vi "Editor.vi"(8 "error in (no error)":errorcluster, 10 "Browse start path":path caption="start path") -> (0 "error out":errorcluster, 3 "Uncompiled sequence out":T2[](array[typedef]))   [LabVIEW 2020, in "Sequencer.lvlib"]
doc: "Sequence editor used to configure, save and load sequences put together of messages."
uses:
  Sequencer.lvlib
  Controls/Ctl_SequenceElement.ctl
  Controls/Ctl_SequenceControlElement.ctl
  PPL/HDH.Actor Framework.Core.Msg.lvlibp/Flex Msg/Controls/Ctl_Control Element.ctl
  Controls/Ctl_MessageListElement.ctl
  PPL/HDH.Actor Framework.Core.Msg.lvlibp/Flex Msg/Flex Msg.lvclass
  PPL/HDH.Actor Framework.Core.Msg.lvlibp
panel:
  in  "Refresh Class List":bool
  in  "Tab Control":T1(tab)
  in  "Message List":i32(listbox)
  in  "Hierarchy Tree":string(tree)
  in  "Search List":i32(listbox)
  in  "Message Filter":string
  in  "Load":bool
  in  "Save":bool
  in  "Append":bool
  in  "Insert":bool
  in  "Sequence":i32[](listbox)
  in  "Empty":bool
  in  "Done":bool
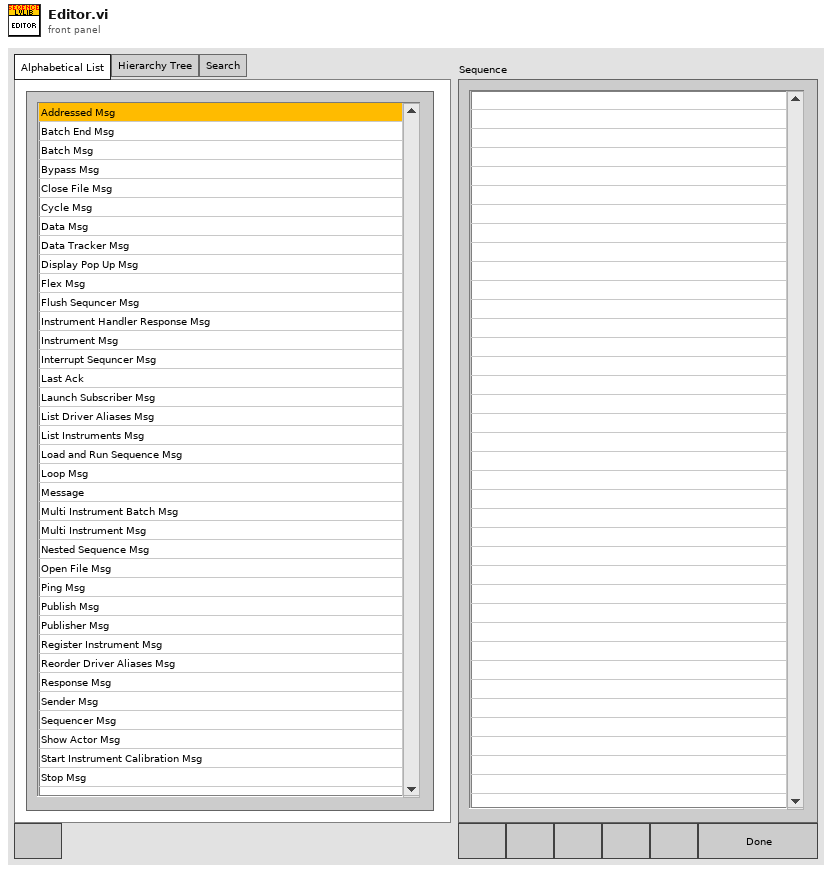
[diagram p1: front panel]
types:
  T1 = enum32{"Alphabetical List", "Hierarchy Tree", "Search"}
  T2 = typedef "Sequencer.lvlib/Ctl_SequenceElement.ctl" = cluster{"Message Base Name":string, "Message Path":path, "Supports Data Access?":bool, "List Symbol":i32, "Sequence Control Element Array":T3[]}
  T3 = typedef "Sequencer.lvlib/Ctl_SequenceControlElement.ctl" = cluster{"Data Override name":string, "Looped Override?":bool, "Control element":T4, "List Symbol":i32}
  T4 = typedef "HDH.Actor Framework.Core.Msg.lvlibp/Ctl_Control Element.ctl" = cluster{"Index":i32, "Label":string, "Value":variant}
  T5 = typedef "Sequencer.lvlib/Ctl_MessageListElement.ctl" = cluster{"Base Name":string, "List index":i32, "Msg path":path, "Supports DA?":bool, "Symbol":i32}
  T6 = typedef "eventvkey.ctl" = enum16{"ASCII", "Enter", "Return", "Shift", "Ctrl", "Alt", "Cmd", "Opt", "Caps", "NumLock", "Clear", "Break", "Up", "Down", "Left", "Right", "Insert", "Delete", "Home", "End", "PageUp", "PageDown", "Escape", "Help", "Pause", "ScrollLock", "F1", "F2", "F3", "F4", "F5", "F6", "F7", "F8", "F9", "F10", "F11", "F12", "F13", "F14", "F15", "F16", "F17", "F18", "F19", "F20", "F21", "F22", "F23", "F24", "Play", "VolumeUp", "VolumeDown", "Mute", "Two Byte Char"}
  T7 = typedef "lveventtype.ctl" = enum32{"Null", "Timeout", "Annotation Menu Selection", "Annotation Menu Selection?", "App Instance Close", "App Instance Close?", "Autoscale Range Change", "Bookmark Info Change", "Cell Edit", "Cell Edit?", "Cursor Grab", "Cursor Grab?", "Cursor Menu Selection", "Cursor Menu Selection?", "Cursor Move", "Cursor Release", "Data Change", "Direction Change", "Display State Change", "Drag Ended", "Drag Enter", "Drag Leave", "Drag Over", "Drag Source Update", "Drag Starting", "Drag Starting?", "Drop", "Exec State Change", "Key Down", "Key Down?", "Key Repeat", "Key Repeat?", "Key Up", "Listbox Double Click", "Menu Activation?", "Menu Selection (App)", "Menu Selection? (App)", "Menu Selection (User)", "Mouse Down", "Mouse Down?", "Mouse Enter", "Mouse Leave", "Mouse Move", "Mouse Up", "Mouse Wheel", "NI Security User Change (App)", "Pane Size", "Panel Close", "Panel Close?", "Panel Resize", "Plot Attribute Change", "Scale Range Change", "Shortcut Menu Activation?", "Shortcut Menu Selection (App)", "Shortcut Menu Selection? (App)", "Shortcut Menu Selection (User)", "Tree Double Click", "Tree Drag", "Tree Drag?", "Tree Drop", "Tree Drop?", "Tree Item Close", "Tree Item Close?", "Tree Item Open", "Tree Item Open?", "User Event", "Value Change"}
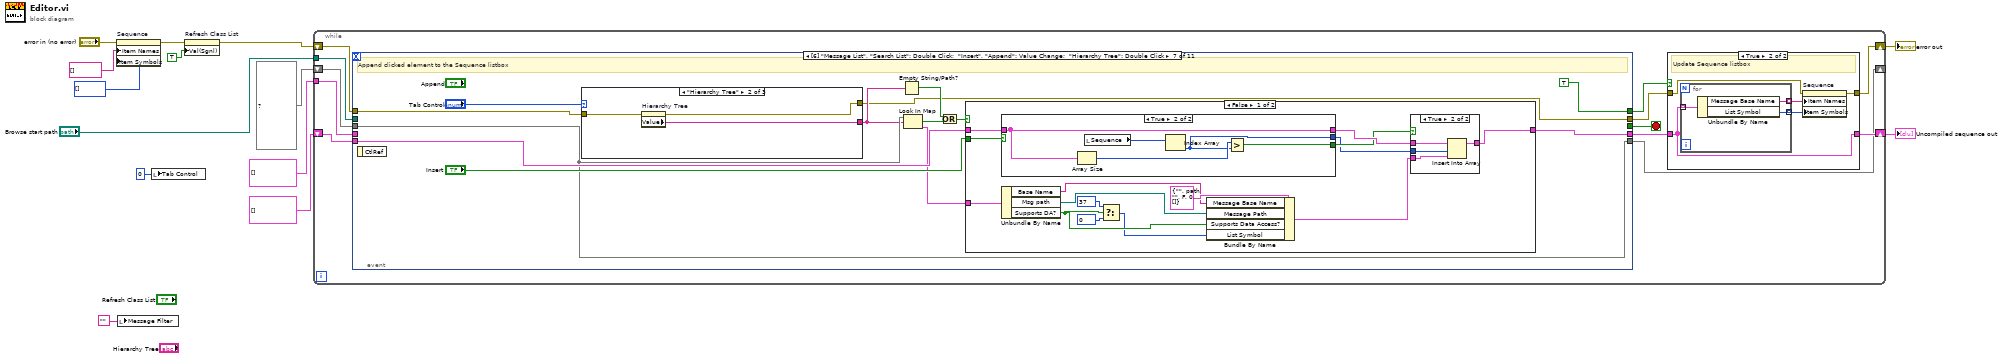
[diagram p0: block diagram]
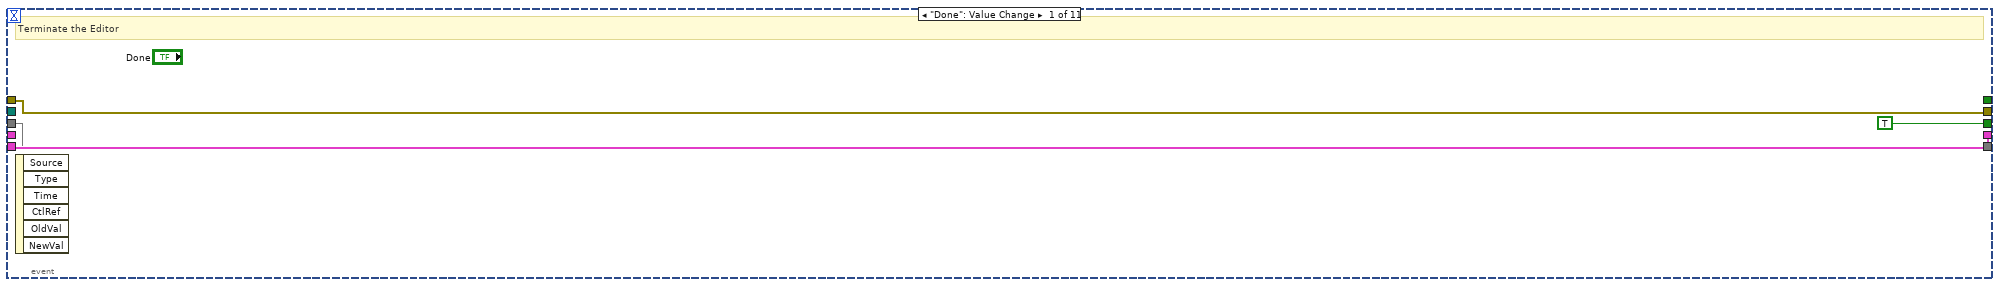
[diagram p3: hidden frame]
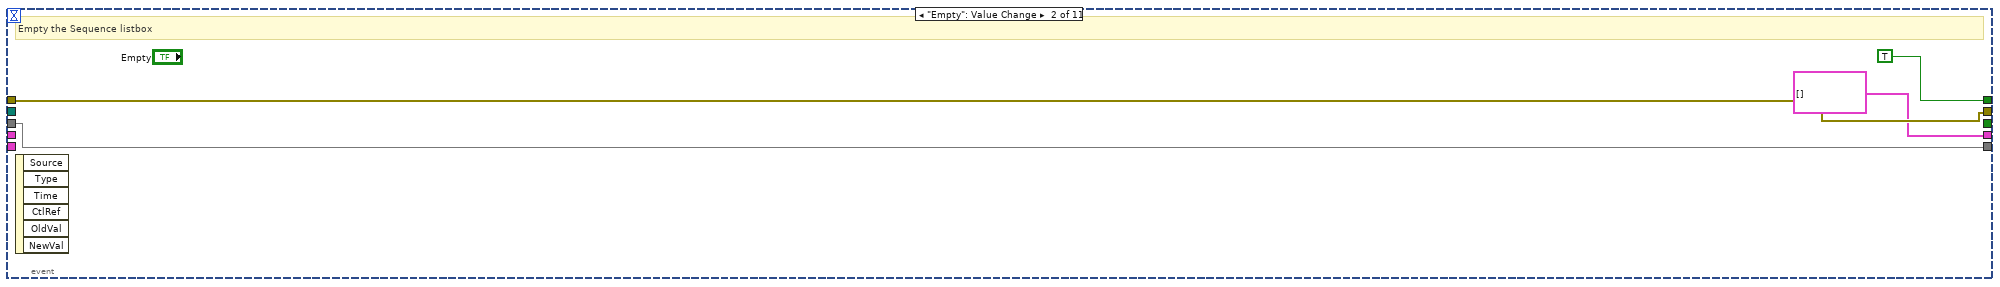
[diagram p4: hidden frame]
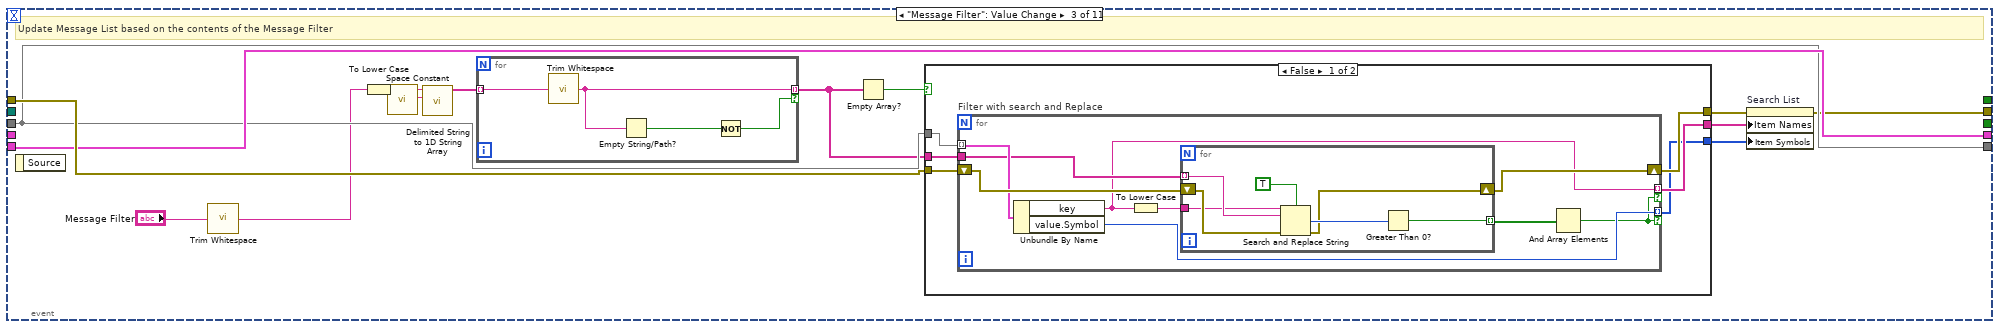
[diagram p5: hidden frame]
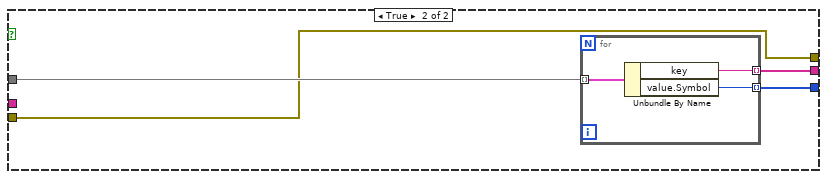
[diagram p6: hidden frame]
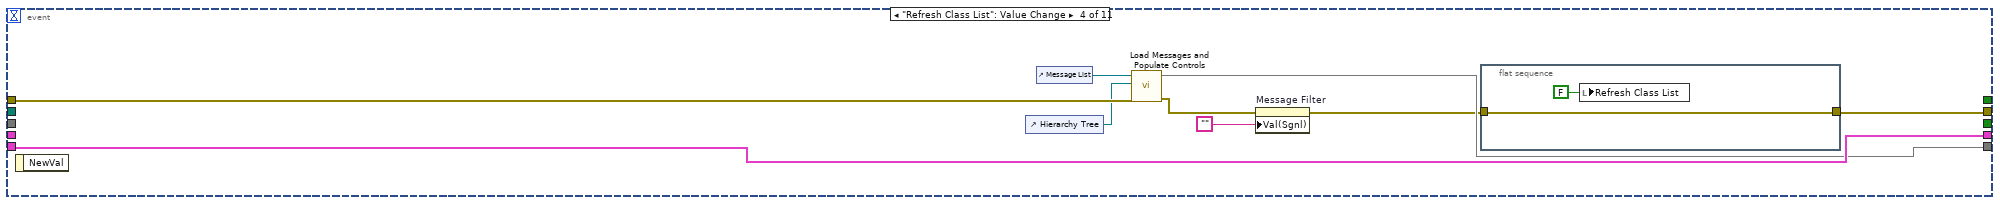
[diagram p7: hidden frame]
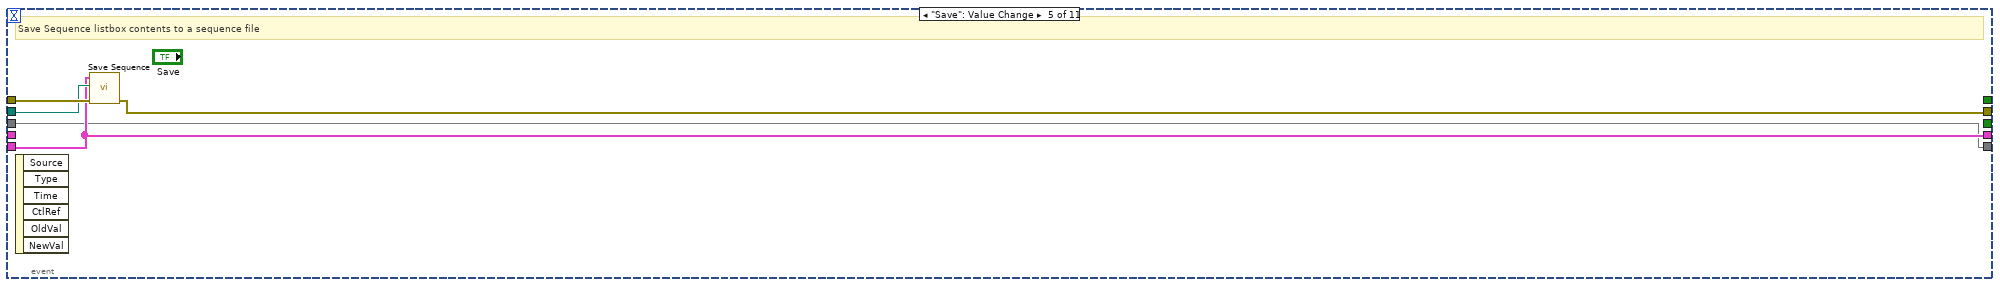
[diagram p8: hidden frame]
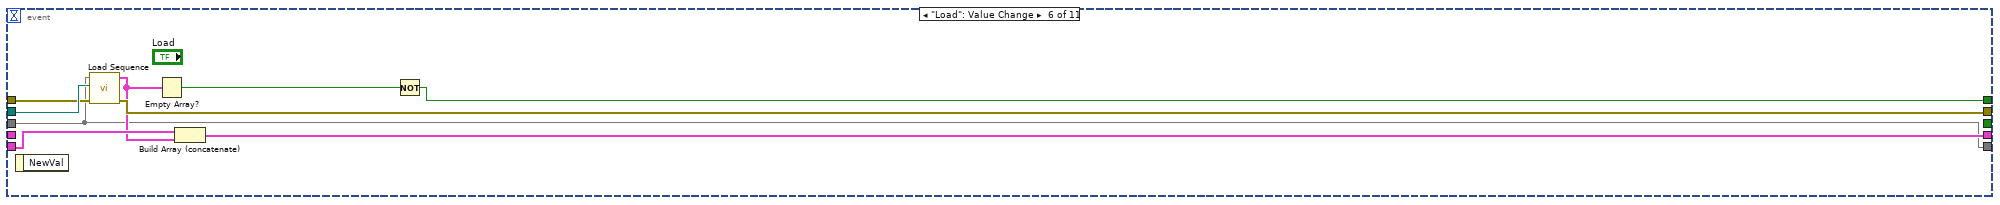
[diagram p9: hidden frame]
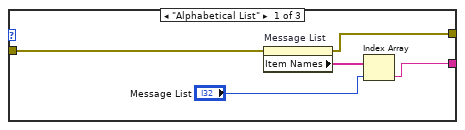
[diagram p10: hidden frame]
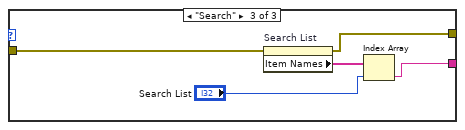
[diagram p11: hidden frame]
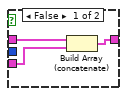
[diagram p12: hidden frame]
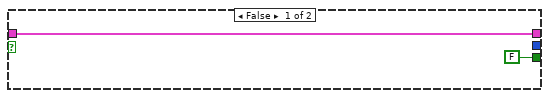
[diagram p13: hidden frame]
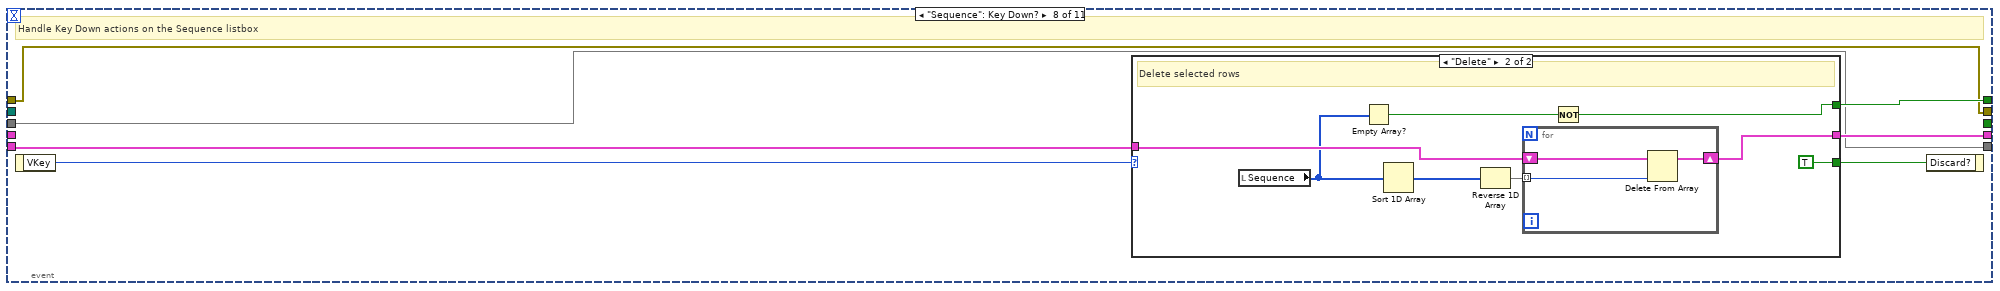
[diagram p15: hidden frame]
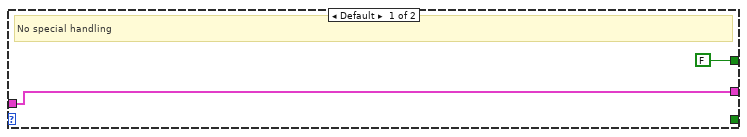
[diagram p16: hidden frame]
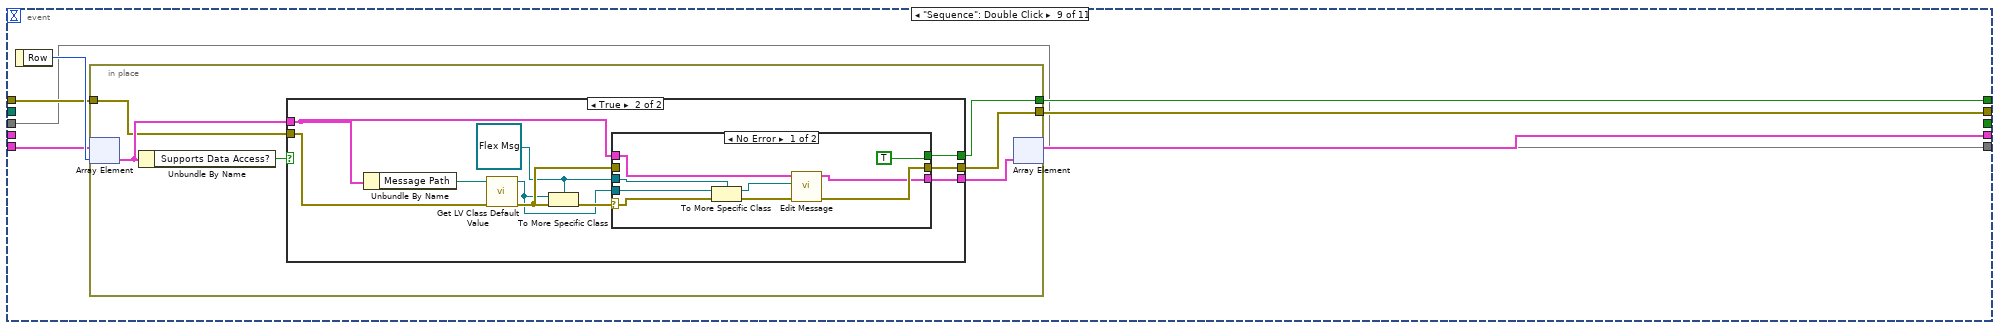
[diagram p17: hidden frame]
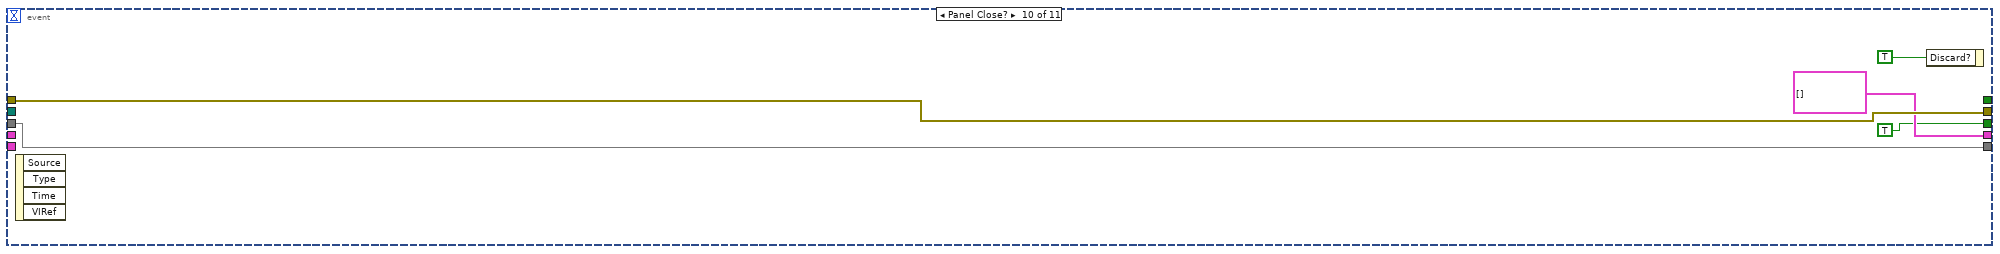
[diagram p20: hidden frame]
diagram:
  n1 = property on="Sequence" class="LstBox (strict)"(error in="error in (no error)", "Item Names"=string[] [], "Item Symbols"=i32[] []) -> (error out=w4:errorcluster)  [unwired: 1 in, 1 out]
  n2 = local write "Message Filter"("") -> ()
  n3 = local write "Tab Control"(u32 0) -> ()
  n4 = property on="Refresh Class List" class="Bool (strict)"(error in=w4, "Val(Sgnl)"=TRUE) -> (error out=w7:errorcluster)  [unwired: 1 in, 1 out]
  n5 = while {
    shift-right: [w19] -> w10
    shift-left: w7 -> [w25]
    shift-right: [w21] -> w11
    shift-left: T2[] [] ("Uncompiled sequence in") -> [w24]
    tunnel: "Browse start path" -> [w18]
    tunnel: T4[] [] ("Control Element Array") -> [w17]
    shift-right: [w15] -> _
    shift-left: map{string, T5} {} ("map") -> [w16]
    stop <- w26 stop-if-true
    n6 = event shown="[6] \"Message List\", \"Search List\": Double Click;  \"Insert\", \"Append\": Value Change;  \"Hierarchy Tree\": Double Click" {
      selector: _ -> [_ _ _ _ _ _ _ _ _ _ _]
      dyn-events: _ -> [_ _ _ _ _ _ _ _ _ _ _]
      timeout: _ -> [_ _ _ _ _ _ _ _ _ _ _]
      tunnel: [TRUE _ _ _ _ _ _ _ _ TRUE _] -> w26
      tunnel: [w39 w44 w53 w99 w106 w112 w118 w174 w195 w233 w243] -> w20
      tunnel: w25 -> [w39 w44 w58 w98 w107 w113 w117 w174 w196 w233 w243]
      tunnel: [w38 T2[] [] ("Uncompiled sequence in") w57 w100 w104 w114 w128 w177 w197 T2[] [] ("Uncompiled sequence in") w237] -> w22
      tunnel: w24 -> [w38 _ w57 w100 w104 w115 w129 w178 w198 _ w238]
      tunnel: [_ TRUE _ _ _ w109 TRUE w176 w194 _ w235] -> w23
      tunnel: w18 -> [_ _ _ _ w105 w116 _ _ _ _ _]
      tunnel: w17 -> [_ _ _ _ _ _ _ _ _ _ _]
      tunnel: w16 -> [w37 w41 w56 _ w103 w108 w124 w173 w193 w229 w234]
      tunnel: [w37 w41 w56 w96 w103 w108 w124 w173 w193 w229 w234] -> w15
      event "Done": Value Change {
        # "Terminate the Editor"
        n7 = event-data() -> ()  [unwired: 1 in, 6 out]
      }
      event "Empty": Value Change {
        # "Empty the Sequence listbox"
        n8 = event-data() -> ()  [unwired: 1 in, 6 out]
      }
      event "Message Filter": Value Change {
        # "Update Message List based on the contents of the Message Filter"
        n9 = event-data() -> ()  [unwired: 1 in, 1 out]
        n10 = call <vilib>:"Trim Whitespace.vi"("string"="Message Filter") -> ("trimmed string"=w52:string)  [unwired: 1 in]
        n11 = To Lower Case(string=w52) -> (all lower case string=w51:string)
        n12 = call <vilib>:"Space Constant.vi"() -> ("String"=w50:string)
        n13 = call <vilib>:"Delimited String to 1D String Array.vi"("delimiter"=w50, "delimited string"=w51) -> ("string array"=w49:string[])  [unwired: 9 in]
        n14 = for {
          tunnel: w49 -> [w62] mode=indexing
          tunnel: [w61] -> w47 mode=indexing if=w59
          n15 = call <vilib>:"Trim Whitespace.vi"("string"=w62) -> ("trimmed string"=w61:string)  [unwired: 1 in]
          n16 = Empty String/Path?(string/path=w61) -> (empty?=w60:bool)
          n17 = Not(x=w60) -> (.not. x?=w59:bool)
        }
        n18 = Empty Array?(array=w47) -> (empty?=w48:bool)
        n19 = case shown="False" w48 {
          tunnel: [w67 w85] -> w46
          tunnel: w58 -> [w68 w85]
          tunnel: w56 -> [w66 w88]
          tunnel: [w64 w87] -> w55
          tunnel: [w63 w86] -> w54
          tunnel: w47 -> [w65 _]
          frame False {
            n20 = for "Filter with search and Replace" {
              tunnel: w66 -> [w76] mode=indexing
              tunnel: [w71] -> w64 mode=indexing if=w69
              shift-right: [w74] -> w67
              shift-left: w68 -> [w77]
              tunnel: w65 -> [w72]
              tunnel: [w70] -> w63 mode=indexing if=w69
              n21 = Unbundle By Name(w76) -> ("key"=w71:string, "value.Symbol"=w70:i32)
              n22 = To Lower Case(string=w71) -> (all lower case string=w73:string)
              n23 = for {
                tunnel: w72 -> [w83] mode=indexing
                tunnel: [w80] -> w75 mode=indexing
                tunnel: w73 -> [w78]
                shift-right: [w79] -> w74
                shift-left: w77 -> [w84]
                n24 = Search and Replace String(case sensitive?=TRUE ("ignore case? (F)"), input string=w78, search string=w83, error in=w84) -> (number of replacements=w81:i32, error out=w79:errorcluster)  [unwired: 4 in, 2 out]
                n25 = Greater Than 0?(x=w81) -> (x > 0?=w80:bool)
              }
              n26 = And Array Elements(Boolean array=w75) -> (logical AND=w69:bool)
            }
          }
          frame True {
            n27 = for {
              tunnel: w88 -> [w91] mode=indexing
              tunnel: [w90] -> w87 mode=indexing
              tunnel: [w89] -> w86 mode=indexing
              n28 = Unbundle By Name(w91) -> ("key"=w90:string, "value.Symbol"=w89:i32)
            }
          }
        }
        n29 = property on="Search List" class="LstBox (strict)"(error in=w46, "Item Names"=w55, "Item Symbols"=w54) -> (error out=w53:errorcluster)  [unwired: 1 in, 1 out]
      }
      event "Refresh Class List": Value Change {
        n30 = event-data() -> ()  [unwired: 1 in, 1 out]
        n31 = control-ref of="Hierarchy Tree"() -> (w95:refnum<vi>)
        n32 = control-ref of="Message List"() -> (w97:refnum<vi>)
        n33 = call "Load Messages and Populate Controls.vi"("error in (no error)"=w98, "Hierarchy"=w95, "ListBox in"=w97) -> ("error out"=w93:errorcluster, "Message map"=w96:map{string, T5})  [unwired: 7 in]
        n34 = property on="Message Filter" class="Str"(error in=w93, "Val(Sgnl)"="") -> (error out=w92:errorcluster)  [unwired: 1 in, 1 out]
        n35 = flat-sequence {
          tunnel: [w102] -> w99
          tunnel: w92 -> [w102]
          frame #0 {
            n36 = local write "Refresh Class List"(FALSE) -> ()
          }
        }
      }
      event "Save": Value Change {
        # "Save Sequence listbox contents to a sequence file"
        n37 = event-data() -> ()  [unwired: 1 in, 6 out]
        n38 = call "Save Sequence.vi"("error in (no error)"=w107, "Browse start path"=w105, "Uncompiled sequence in"=w104) -> ("error out"=w106:errorcluster)  [unwired: 8 in]
      }
      event "Load": Value Change {
        n39 = event-data() -> ()  [unwired: 1 in, 1 out]
        n40 = call "Load Sequence.vi"("error in (no error)"=w113, "Browse path"=w116, "Message map"=w108) -> ("error out"=w112:errorcluster, "Uncompiled Sequence out"=w111:T2[])  [unwired: 7 in]
        n41 = Empty Array?(array=w111) -> (empty?=w110:bool)
        n42 = Build Array (concatenate)(w115, w111) -> (w114:T2[])
        n43 = Not(x=w110) -> (.not. x?=w109:bool)
      }
      event "Message List", "Hierarchy Tree", "Search List": Double Click; "Insert", "Append": Value Change {
        # "Append clicked element to the Sequence listbox"
        n44 = event-data() -> ()  [unwired: 1 in, 1 out]
        n45 = case shown="\"Hierarchy Tree\"" "Tab Control" {
          tunnel: [w132 w137 w140] -> w123
          tunnel: w117 -> [w131 w136 w139]
          tunnel: [w130 w135 w138] -> w118
          frame "Alphabetical List" {
            n46 = property on="Message List" class="LstBox (strict)"(error in=w131) -> (error out=w130:errorcluster, "Item Names"=w134:string[])  [unwired: 1 in, 1 out]
            n47 = Index Array(array=w134, index="Message List") -> (element=w132:string)
          }
          frame "Hierarchy Tree" {
            n48 = property on="Hierarchy Tree" class="Tree (strict)"(error in=w136) -> (error out=w135:errorcluster, "Value"=w137:string)  [unwired: 1 in, 1 out]
          }
          frame "Search" {
            n49 = property on="Search List" class="LstBox (strict)"(error in=w139) -> (error out=w138:errorcluster, "Item Names"=w142:string[])  [unwired: 1 in, 1 out]
            n50 = Index Array(array=w142, index="Search List") -> (element=w140:string)
          }
        }
        n51 = Empty String/Path?(string/path=w123) -> (empty?=w121:bool)
        n52 = Look In Map(map=w124, key=w123) -> (key not found?=w122:bool, value=w119:T5)  [unwired: 1 in]
        n53 = Or(x=w121, y=w122) -> (x .or. y?=w120:bool)
        n54 = case shown="False" w120 {
          tunnel: [w148 w172] -> w128
          tunnel: w129 -> [w146 w172]
          tunnel: w119 -> [w157 _]
          tunnel: "Insert" -> [w147 _]
          frame False {
            n55 = case shown="True" w147 {
              tunnel: w146 -> [w166 w170]
              tunnel: [w166 w170] -> w145
              tunnel: [FALSE w168] -> w144
              tunnel: [_ w167] -> w143
              frame False {
              }
              frame True {
                n56 = Array Size(array=w170) -> (size(s)=w169:i32)
                n57 = local read "Sequence"() -> (w171:i32[])
                n58 = Index Array(array=w171) -> (element=w167:i32)  [unwired: 1 in]
                n59 = Greater?(x=w169, y=w167) -> (0:w168:bool)
              }
            }
            n60 = Unbundle By Name(w157) -> ("Base Name"=w155:string, "Msg path"=w154:path, "Supports DA?"=w153:bool)
            n61 = Select(t=37, s=w153, f=0) -> (s? t:f=w150:i32)
            n62 = Bundle By Name(cluster=T2 {"Message Base Name"="", "Message Path"=path "", "Supports Data Access?"=FALSE, "List Symbol"=0, "Sequence Control Element Array"=[]} ("Uncompiled sequence in"), "Message Base Name"=w155, "Message Path"=w154, "Supports Data Access?"=w153, "List Symbol"=w150) -> (w149:T2)
            n63 = case shown="True" w144 {
              tunnel: w149 -> [w160 w163]
              tunnel: [w159 w161] -> w148
              tunnel: w145 -> [w158 w164]
              tunnel: w143 -> [_ w162]
              frame False {
                n64 = Build Array (concatenate)(w158, w160) -> (w159:T2[])
              }
              frame True {
                n65 = Insert Into Array(array=w164, index=w162, new element=w163) -> (w161:T2[])
              }
            }
          }
          frame True {
          }
        }
      }
      event "Sequence": Key Down? {
        # "Handle Key Down actions on the Sequence listbox"
        n66 = event-data() -> ("VKey"=w179:T6)  [unwired: 1 in]
        n67 = case shown="\"Delete\"" w179 {
          tunnel: w178 -> [w181 w189]
          tunnel: [w181 w188] -> w177
          tunnel: [FALSE w182] -> w176
          tunnel: [_ TRUE ("Discard?")] -> w175
          frame Default {
            # "No special handling"
          }
          frame "Delete" {
            # "Delete selected rows"
            n68 = local read "Sequence"() -> (w184:i32[])
            n69 = Empty Array?(array=w184) -> (empty?=w183:bool)
            n70 = Sort 1D Array(array=w184) -> (sorted array=w186:i32[])
            n71 = Reverse 1D Array(array=w186) -> (reversed array=w185:i32[])
            n72 = for {
              shift-right: [w191] -> w188
              shift-left: w189 -> [w192]
              tunnel: w185 -> [w190] mode=indexing
              n73 = Delete From Array(array=w192, index=w190) -> (array with subset deleted=w191:T2[])  [unwired: 1 in, 1 out]
            }
            n74 = Not(x=w183) -> (.not. x?=w182:bool)
          }
        }
        n75 = event-data("Discard?"=w175) -> ()  [unwired: 1 in, 1 out]
      }
      event "Sequence": Double Click {
        n76 = event-data() -> ("Row"=w199:i32)  [unwired: 1 in]
        n77 = in-place {
          in-place-border: w196 -> [w202]
          in-place-border: [w201] -> w195
          in-place-border: [w200] -> w194
          n78 = in-place-array #1(w198, w199) -> (w203:T2)
          n79 = Unbundle By Name(w203) -> ("Supports Data Access?"=w205:bool)
          n80 = case shown="True" w205 {
            tunnel: [w207 w214] -> w204
            tunnel: w203 -> [w207 w213]
            tunnel: w202 -> [w206 w216]
            tunnel: [w206 w212] -> w201
            tunnel: [_ w208] -> w200
            frame False {
            }
            frame True {
              w209 = refnum<class "Flex Msg.lvclass"> refnum ("HDH.Actor Framework.Core.Msg.lvlibp:Flex Msg.lvclass")
              n81 = Unbundle By Name(w213) -> ("Message Path"=w217:path)
              n82 = call <vilib>:"Get LV Class Default Value.vi"("error in (no error)"=w216, "class path"=w217) -> ("error out"=w211:errorcluster, "object"=w210:refnum<class>)  [unwired: 8 in]
              n83 = To More Specific Class(target class=w209, reference=w210, error in=w211) -> (error out=w215:errorcluster)  [unwired: 1 out]
              n84 = case shown="No Error" w215 {
                selector: w215 -> [w226 _]
                tunnel: [w222 w228] -> w214
                tunnel: w213 -> [w221 w228]
                tunnel: [w223 w227] -> w212
                tunnel: w211 -> [_ w227]
                tunnel: w210 -> [w225 _]
                tunnel: w209 -> [w224 _]
                tunnel: [TRUE _] -> w208
                frame No Error {
                  n85 = To More Specific Class(target class=w224, reference=w225, error in=w226) -> (specific class reference=w220:refnum<class "Flex Msg.lvclass">, error out=w219:errorcluster)
                  n86 = call "Edit Message.vi"("error in (no error)"=w219, "Flex Msg in"=w220, "Sequence Element in"=w221) -> ("error out"=w223:errorcluster, "Sequence Element out"=w222:T2)  [unwired: 7 in]
                }
                frame Error {
                }
              }
            }
          }
          n87 = in-place-array #1(w204) -> (w197:T2[])  [unwired: 1 out]
        }
      }
      event Panel Close? {
        n88 = event-data() -> ()  [unwired: 1 in, 4 out]
        n89 = event-data("Discard?"=TRUE) -> ()  [unwired: 1 in, 1 out]
      }
      event "Sequence": Drag Starting; "Sequence": Drag Ended {
        w236 = i32[] []
        # "Handle drag and drop in the sequence listbox"
        n90 = event-data() -> ("Type"=w241:T7)  [unwired: 1 in]
        n91 = feedback #2(w236) -> (w239:i32[])
        n92 = case shown="\"Drag Ended\"" w241 {
          tunnel: "Sequence" -> [_ w248 w261]
          tunnel: [w244 w247 w249] -> w240
          tunnel: w239 -> [_ _ w254]
          tunnel: w238 -> [w245 w246 w253]
          tunnel: [w245 w246 w252] -> w237
          tunnel: [_ _ TRUE] -> w235
          tunnel: w236 -> [w244 _ w249]
          frame Default {
          }
          frame "Drag Starting" {
            n93 = To Long Integer(number=w248) -> (32bit integer=w247:i32[])
          }
          frame "Drag Ended" {
            n94 = Reverse 1D Array(array=w254) -> (reversed array=w260:i32[])
            n95 = Index Array(array=w261) -> (element=w250:i32)  [unwired: 1 in]
            n96 = for {
              tunnel: w260 -> [w271] mode=indexing
              shift-right: [w270] -> w255
              shift-left: w253 -> [w272]
              tunnel: [w269] -> w259 mode=indexing
              n97 = Delete From Array(array=w272, index=w271) -> (deleted portion=w269:T2, array with subset deleted=w270:T2[])  [unwired: 1 in]
            }
            n98 = Array Size(array=w255) -> (size(s)=w257:i32)
            n99 = Reverse 1D Array(array=w259) -> (reversed array=w258:T2[])
            n100 = Greater?(x=w257, y=w250) -> (0:w256:bool)
            n101 = case shown="True" w256 {
              tunnel: w255 -> [w264 w268]
              tunnel: [w262 w267] -> w252
              tunnel: w258 -> [w263 w266]
              tunnel: w250 -> [_ w265]
              frame False {
                n102 = Build Array (concatenate)(w264, w263) -> (w262:T2[])
              }
              frame True {
                n103 = Insert Into Array(array=w268, index=w265, new element=w266) -> (w267:T2[])
              }
            }
          }
        }
        n104 = feedback-in #2(w240) -> ()
      }
    }
    n105 = case shown="True" w23 {
      tunnel: w22 -> [w28 w33]
      tunnel: [w28 w33] -> w21
      tunnel: w20 -> [w27 w30]
      tunnel: [w27 w29] -> w19
      frame False {
      }
      frame True {
        # "Update Sequence listbox"
        n106 = for {
          tunnel: w33 -> [w36] mode=indexing
          tunnel: [w35] -> w32 mode=indexing
          tunnel: [w34] -> w31 mode=indexing
          n107 = Unbundle By Name(w36) -> ("Message Base Name"=w35:string, "List Symbol"=w34:i32)
        }
        n108 = property on="Sequence" class="LstBox (strict)"(error in=w30, "Item Names"=w32, "Item Symbols"=w31) -> (error out=w29:errorcluster)  [unwired: 1 in, 1 out]
      }
    }
  }
  "Uncompiled sequence out" <- w11
  "error out" <- w10
